vi "CropAndCombineTIFFs_list.vi"() -> ()   [LabVIEW 2011]
uses:
  tiff/TiffModules/AddTiffPage_U16_text_res.vi
panel:
  in  "BigTiff,Endian":u16(ring)=257 items=["Big-Endian"=0, "Native"=1, "Little-Endian"=2, "BigTiff-Big-Endian"=256, "Bigtiff,Native"=257, "Biftiff,Littleendian"=258]
  in  "Stop at offset:":u64=429496729500
  out "Input-File":i32
  out "AfterDIRoffset":u64 format="%09d"
  in  "Files":path[](array[path])
  in  "y-length":i32=1040
  in  "y-start":i32
  in  "x-length":i32=2286
  in  "x-start":i32
  out "Input-page":i32
  out "string":string
  out "xy-resolution":cluster{"x":dbl, "y":dbl}
  out "Out":u16[][](graph)
  out "In":u16[][](graph)
  # "select all tiff files, with correct order!\nenter crop data (wie IJ!)\nrun\nnew name first with _cropcombine.tif\nstops at max tiff-offset 2^32"
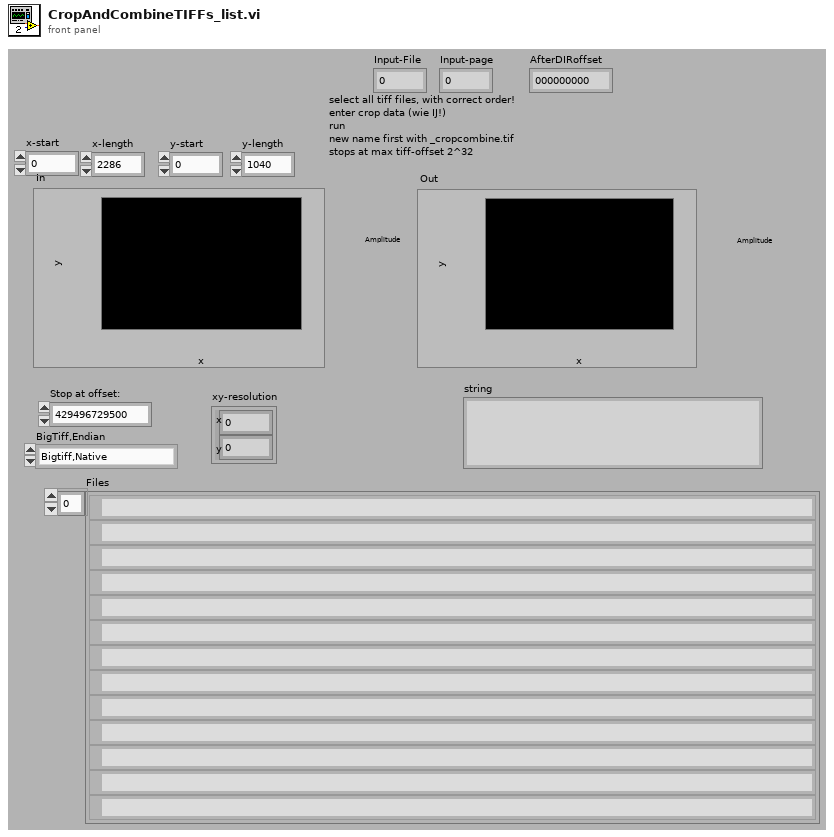
[diagram p1: front panel]
types:
  T1 = cluster{"Tiff refnum":refnum<file>, "BigTiff,Endian":u16}
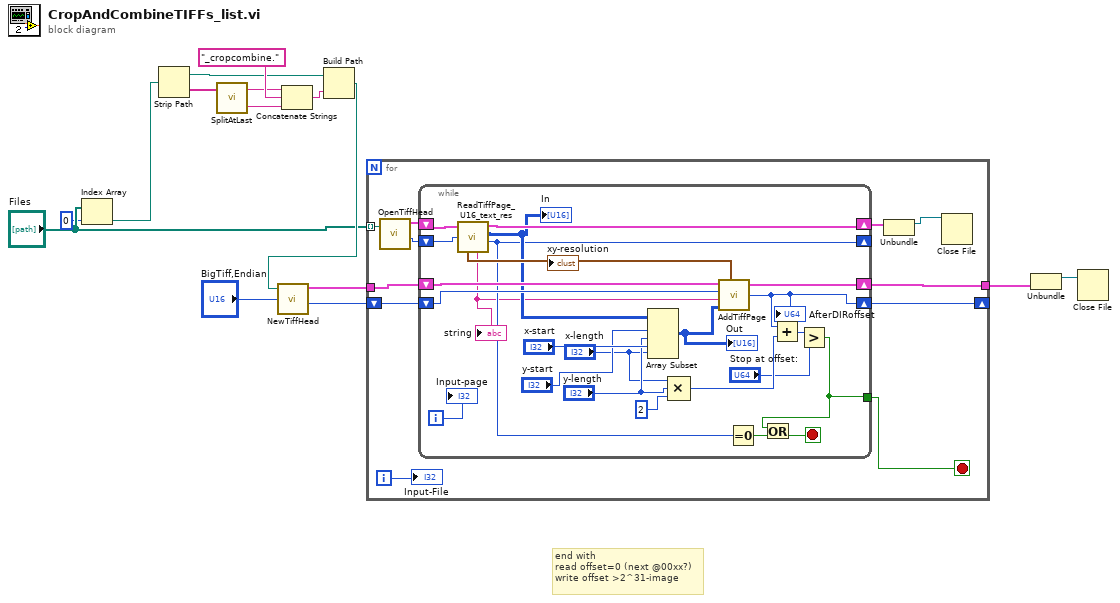
[diagram p0: block diagram]
diagram:
  # "end with \nread offset=0 (next @00xx?)\nwrite offset >2^31-image"
  n1 = Index Array(array="Files", index=0) -> (element=w2:path)
  n2 = Strip Path(path=w2) -> (stripped path=w5:path, name=w6:string)
  n3 = call "SplitAtLast.vi"("In-String"=w6) -> ("end"=w14:string, "Front (default)"=w7:string)  [unwired: 1 in]
  n4 = Concatenate Strings(w7, "_cropcombine." ("String"), w14) -> (w13:string)
  n5 = Build Path(base path=w5, name or relative path=w13) -> (appended path=w12:path)
  n6 = call "NewTiffHead.vi"("file path"=w12, "BigTiff,Endian"="BigTiff,Endian") -> ("TIFF file"=w11:T1, "Place for first IFD (8,eof-position)"=w10:u64)  [unwired: 2 in, 1 out]
  n7 = for {
    tunnel: w11 -> [w25]
    tunnel: [w21] -> w9
    tunnel: "Files" -> [w19] mode=indexing
    shift-right: [w16] -> _
    shift-left: w10 -> [w23]
    i -> [w17]
    stop <- w18 stop-if-true
    n8 = call "OpenTiffHead.vi"("file path"=w19) -> ("TIFF file"=w26:T1, "first Diroffset"=w24:u64)  [unwired: 2 in, 1 out]
    n9 = while {
      shift-right: [w41] -> w22
      shift-left: w26 -> [w44]
      shift-right: [w49] -> w21
      shift-left: w25 -> [w50]
      shift-right: [w39] -> _
      shift-left: w24 -> [w43]
      shift-right: [w32] -> w16
      shift-left: w23 -> [w48]
      tunnel: [w27] -> w18
      i -> [w46]
      stop <- w28 stop-if-true
      n10 = call "ReadTiffPage_U16_text_res.vi"("TIFF file"=w44, "IFDoffset"=w43) -> ("Pixelsize [µm]"=w42:cluster{"x":dbl, "y":dbl}, "TIFF file out"=w41:T1, "16-bit pixmap"=w40:u16[][], "string"=w38:string, "Next offset"=w39:i64)  [unwired: 3 in, 1 out]
      "In" <- w40
      "xy-resolution" <- w42
      "string" <- w38
      n11 = Array Subset(array=w40, index (row)="y-start", length (row)="y-length", index (col)="x-start", length (col)="x-length") -> (w45:u16[][])
      "Out" <- w45
      n12 = Compound Arithmetic op=MULTIPLY("x-length", "y-length", u64 2 ("value")) -> (w31:u64)
      n13 = call-poly "AddTiffPage.vi"("TIFF file"=w50, "After last DIROffset"=w48, "Text"=w38, "16-bit pixmap x, y"=w45, "Pixelsize [µm]"=w42) -> ("TIFF file"=w49:T1, "AfterDIRoffset"=w32:u64)  [unwired: 1 out]
      "AfterDIRoffset" <- w32
      n14 = Equal To 0?(x=w39) -> (x = 0?=w47:bool)
      n15 = Add(x=w32, y=w31) -> (x+y=w30:u64)
      n16 = Greater?(x=w30, y="Stop at offset:") -> (0:w27:bool)
      n17 = Or(x=w27, y=w47) -> (x .or. y?=w28:bool)
      "Input-page" <- w46
    }
    n18 = Unbundle(w22) -> ("Tiff refnum"=w20:refnum<file>)  [unwired: 1 out]
    n19 = Close File(refnum=w20) -> ()  [unwired: 1 in, 2 out]
    "Input-File" <- w17
  }
  n20 = Unbundle(w9) -> ("Tiff refnum"=w8:refnum<file>)  [unwired: 1 out]
  n21 = Close File(refnum=w8) -> ()  [unwired: 1 in, 2 out]
